vi "Read setSpectTempSetpoint.vi"(8 "error in (no error)":errorcluster, 11 "setSpectTempSetpoint in":refnum<class "setSpectTempSetpoint.lvclass">) -> (0 "error out":errorcluster, 2 "command_setSpectTempSetpoint":T1, 3 "setSpectTempSetpoint out":refnum<class "setSpectTempSetpoint.lvclass">)   [LabVIEW 2016, in "Commands.lvlib" / "setSpectTempSetpoint.lvclass"]
uses:
  setSpectTempSetpoint.lvclass
  ts_sallv_sedspectrometer/DataTypes/command_setSpectTempSetpoint.ctl
  setSpectTempSetpoint.lvclass/setSpectTempSetpoint.ctl
  ts_sallv_sedspectrometer/SALLV_sedSpectrometer.lvlib
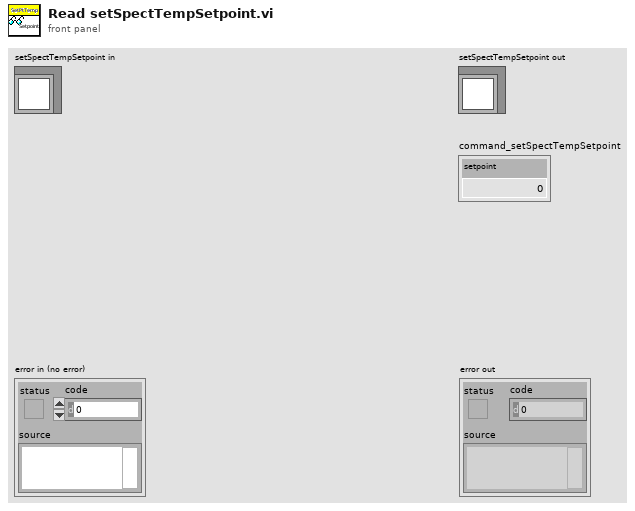
[diagram p1: front panel]
types:
  T1 = typedef "SALLV_sedSpectrometer.lvlib/command_setSpectTempSetpoint.ctl" = cluster{"setpoint":sgl}
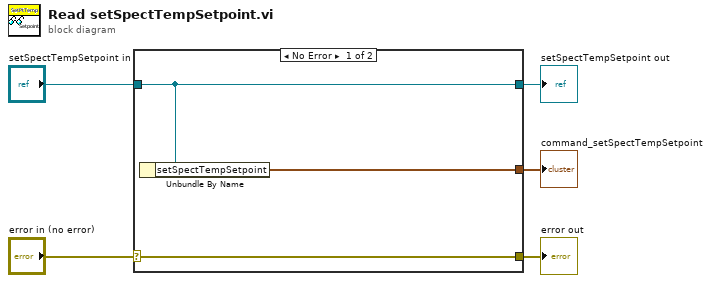
[diagram p0: block diagram]
diagram:
  n1 = case shown="No Error" "error in (no error)" {
    selector: "error in (no error)" -> [w8 w9]
    tunnel: [w8 w9] -> w4
    tunnel: [w7 w10] -> w2
    tunnel: "setSpectTempSetpoint in" -> [w7 w10]
    tunnel: [w6 _] -> w1
    frame No Error {
      n2 = Unbundle By Name(w7) -> ("setSpectTempSetpoint"=w6:T1)
    }
    frame Error {
    }
  }
  "error out" <- w4
  "setSpectTempSetpoint out" <- w2
  "command_setSpectTempSetpoint" <- w1
